vi "Initialize HW.vi"(8 "error in (no error)":errorcluster, 11 "USB Camera in":refnum<class "USB Camera.lvclass">) -> (0 "error out":errorcluster, 3 "USB Camera out":refnum<class "USB Camera.lvclass">)   [LabVIEW 2020, in "USB Camera.lvclass"]
uses:
  USB Camera.lvclass
  USB Camera.lvclass/USB Camera.ctl
  Camera.lvclass
  <vilib>/vision/driver/NI_Vision_Acquisition_Software.lvlib
panel:
  in  "Settings (Clamp (Rake))":T1
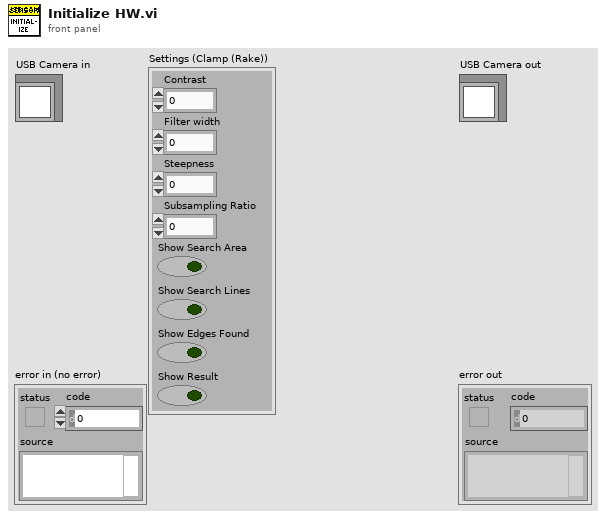
[diagram p1: front panel]
types:
  T1 = cluster{"Contrast":i32, "Filter width":i32, "Steepness":i32, "Subsampling Ratio":u32, "Show Search Area":bool, "Show Search Lines":bool, "Show Edges Found":bool, "Show Result":bool}
  T2 = typedef "Image Type" = u32
  T3 = typedef "IMAQdx.ctl" = refnum<k21>
  T4 = typedef "IMAQ Image.ctl" = refnum<image>
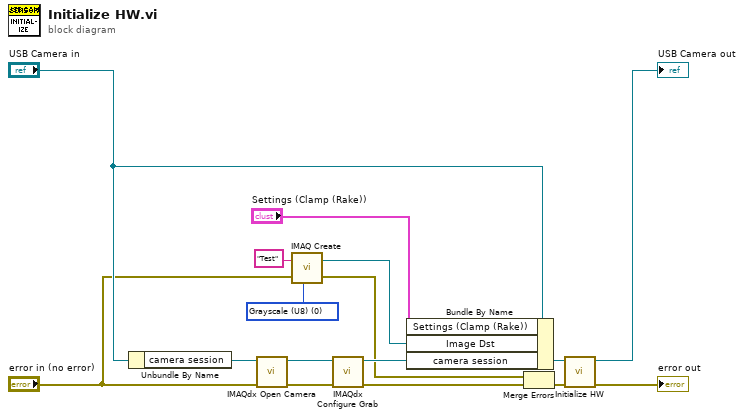
[diagram p0: block diagram]
diagram:
  w7 = T2 0 items=["Grayscale (U8)", "Grayscale (I16)", "Grayscale (SGL)", "Complex (CSG)", "RGB (U32)", "HSL (U32)", "RGB (U64)", "Grayscale (U16)"] ("Image Type")
  n1 = Unbundle By Name("USB Camera in") -> ("camera session"=w14:T3)
  n2 = call <vilib>:"IMAQdx Open Camera.vi"("error in"="error in (no error)", "Session In"=w14) -> ("error out"=w15:errorcluster, "Session Out"=w13:T3)  [unwired: 8 in]
  n3 = call "IMAQ Create"("Image Name"="Test", "Image Type"=w7, "error in (no error)"="error in (no error)") -> ("New Image"=w5:T4, "error out"=w2:errorcluster)  [unwired: 2 in]
  n4 = call <vilib>:"IMAQdx Configure Grab.vi"("error in"=w15, "Session In"=w13) -> ("error out"=w4:errorcluster, "Session Out"=w11:T3)  [unwired: 8 in]
  n5 = Bundle By Name(cluster="USB Camera in", "Settings (Clamp (Rake))"="Settings (Clamp (Rake))", "Image Dst"=w5, "camera session"=w11) -> (w10:refnum<class "USB Camera.lvclass">)
  n6 = Merge Errors(w2, w4) -> (w3:errorcluster)
  n7 = call-parent "Initialize HW.vi"("error in (no error)"=w3, "Camera in"=w10) -> ("error out"=→"error out":errorcluster, "Camera out"=→"USB Camera out":refnum<class "USB Camera.lvclass">)  [unwired: 8 in]
